vi "Remainder_and_Quotient.vi"() -> ()   [LabVIEW 2020]
panel:
  in  "Divisor":dbl
  in  "Dividend":dbl
  out "Quotient":dbl
  out "Remainder":dbl
  # "Divide Two Numbers and Find the Remainder and Quotient."
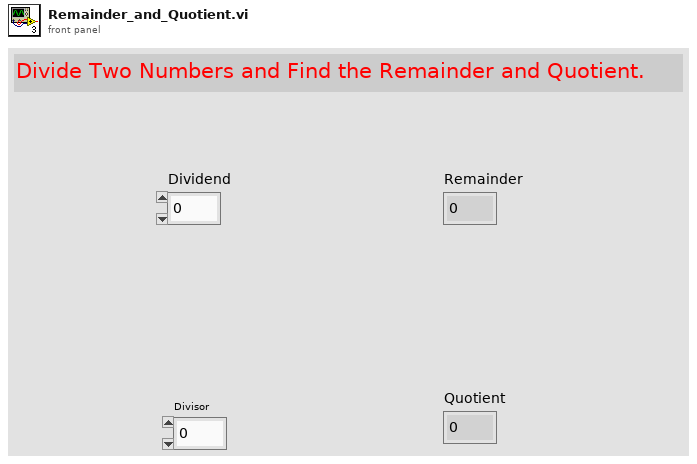
[diagram p1: front panel]
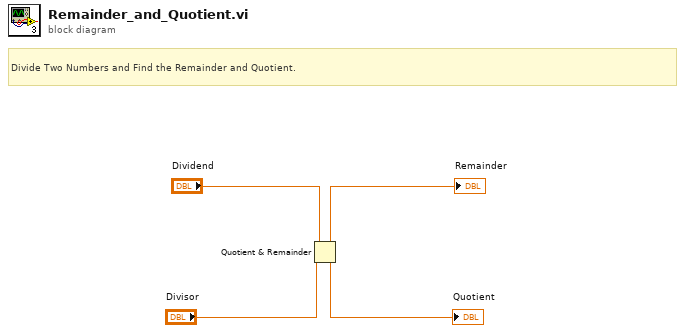
[diagram p0: block diagram]
diagram:
  # "Divide Two Numbers and Find the Remainder and Quotient."
  n1 = Quotient & Remainder(x="Dividend", y="Divisor") -> (x-y*floor(x/y)=→"Remainder":dbl, floor(x/y)=→"Quotient":dbl)
